vi "Delete Instrument Record.vi"(6 "Device":string, 8 "error in":errorcluster, 11 "Config in":refnum<class "Config.lvclass">) -> (0 "error out":errorcluster, 3 "Config out":refnum<class "Config.lvclass">)   [LabVIEW 2023, in "Config.lvlib" / "Config.lvclass"]
doc: "Prompts user to confirm deletion then\nSearches all the sections for the input value (device)\nDeletes the section and all keys within that section from the config file\n****Warning*** this action cannot be undone."
uses:
  Config.lvclass
  Config.lvclass/Config.ctl
  <vilib>/Utility/config.llb/NI_LVConfig.lvlib
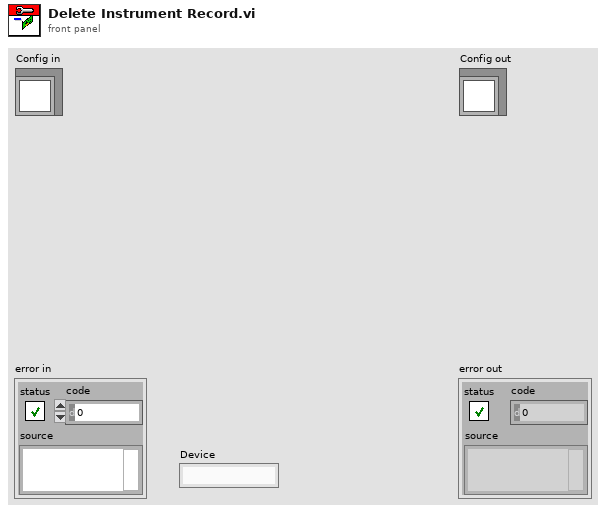
[diagram p1: front panel]
types:
  T1 = typedef "NI_LVConfig.lvlib/Config Data RefNum.ctl" = refnum<k1>
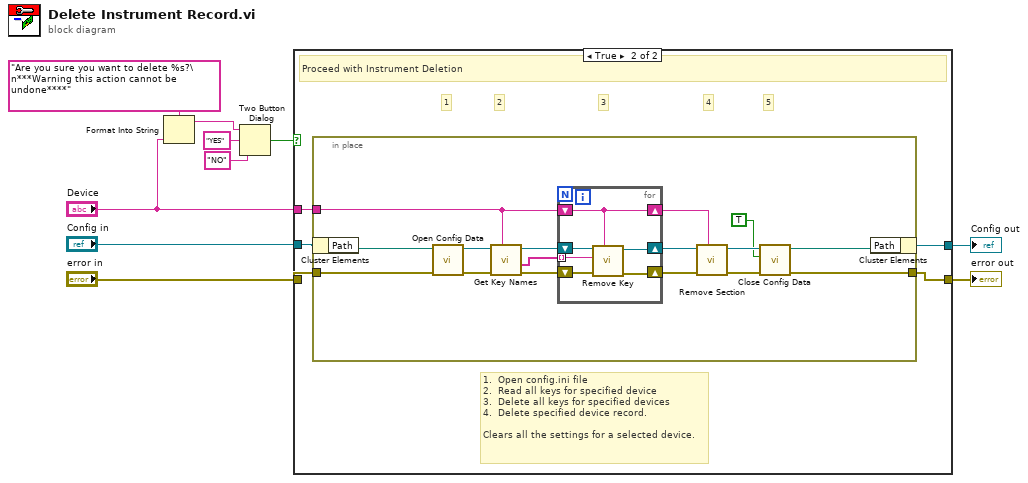
[diagram p0: block diagram]
diagram:
  n1 = Format Into String(format string="Are you sure you want to delete %s?\n***Warning this action cannot be undone****", "Device") -> (resulting string=w3:string)  [unwired: 2 in, 1 out]
  n2 = Two Button Dialog(message=w3, 1:"NO" ("F button name (\"Cancel\")"), 2:"YES" ("T button name (\"OK\")")) -> (T button?=w6:bool)
  n3 = case shown="True" w6 {
    tunnel: "Config in" -> [w12 w17]
    tunnel: [w12 w16] -> w9
    tunnel: "error in" -> [w11 w15]
    tunnel: [w11 w14] -> w7
    tunnel: "Device" -> [_ w13]
    frame False {
      # "Cancel Instrument deletion"
    }
    frame True {
      # "1.  Open config.ini file\n2.  Read all keys for specified device\n3.  Delete all keys for specified devices\n4.  Delete specified device record.\n\nClears all the settings for a selected device."
      # "5"
      # "4"
      # "3"
      # "2"
      # "1"
      # "Proceed with Instrument Deletion"
      n4 = in-place {
        in-place-border: w15 -> [w21]
        in-place-border: [w20] -> w14
        in-place-border: w13 -> [w18]
        n5 = in-place-cluster #1(w17) -> ("Path"=w33:path)
        n6 = call <vilib>:"Open Config Data.vi"("error in (no error)"=w21, "configuration file path"=w33) -> ("error out"=w32:errorcluster, "refnum"=w31:T1)  [unwired: 7 in, 1 out]
        n7 = call <vilib>:"Get Key Names.vi"("section"=w18, "error in (no error)"=w32, "refnum"=w31) -> ("error out"=w30:errorcluster, "key names"=w29:string[], "refnum out"=w28:T1)  [unwired: 5 in, 1 out]
        n8 = for {
          shift-right: [w38] -> w27
          shift-left: w30 -> [w39]
          tunnel: w29 -> [w37] mode=indexing
          shift-right: [w35] -> w26
          shift-left: w28 -> [w36]
          shift-right: [w34] -> w19
          shift-left: w18 -> [w34]
          # "Delete all settings"
          n9 = call <vilib>:"Remove Key.vi"("section"=w34, "error in (no error)"=w39, "key"=w37, "refnum"=w36) -> ("error out"=w38:errorcluster, "refnum out"=w35:T1)  [unwired: 5 in, 1 out]
        }
        n10 = call <vilib>:"Remove Section.vi"("section"=w19, "error in (no error)"=w27, "refnum"=w26) -> ("error out"=w25:errorcluster, "refnum out"=w24:T1)  [unwired: 6 in, 1 out]
        n11 = call <vilib>:"Close Config Data.vi"("error in (no error)"=w25, "write file if changed (T)"=TRUE, "refnum"=w24) -> ("error out"=w20:errorcluster, "file path"=w23:path)  [unwired: 7 in]
        n12 = in-place-cluster #1("Path"=w23) -> (w16:refnum<class "Config.lvclass">)
      }
    }
  }
  "error out" <- w7
  "Config out" <- w9
